vi "Keithley 2400 Source Measuret.vi"(8 "error in (no error)":errorcluster, 10 "Source Settings (Current vs Voltage Source)":T1(ring), 11 "VISA Refnum in":refnum<visa-resource-name>) -> (0 "error out":errorcluster, 3 "Source Value":dbl)   [LabVIEW 2019]
panel:
  # "This gets the value that the source is set\nat from the Keithley 2400\n\nJustin Young\n2012.06.24"
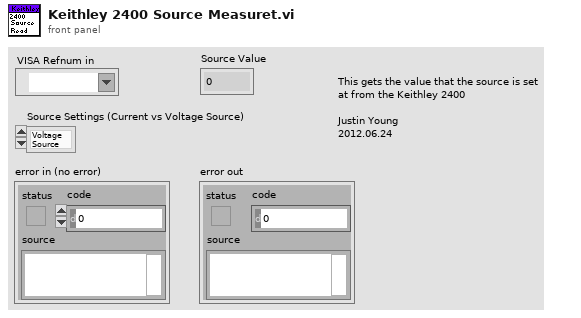
[diagram p1: front panel]
types:
  T1 = enum32{"Voltage Source", "Current Source", "Sense Only"}
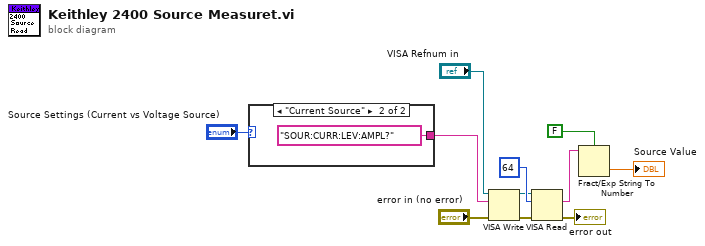
[diagram p0: block diagram]
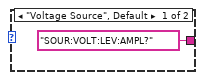
[diagram p2: hidden frame]
diagram:
  n1 = case shown="\"Current Source\"" "Source Settings (Current vs Voltage Source)" {
    tunnel: ["SOUR:VOLT:LEV:AMPL?" ("write buffer") "SOUR:CURR:LEV:AMPL?" ("write buffer")] -> w7
    frame "Voltage Source", Default {
    }
    frame "Current Source" {
    }
  }
  n2 = VISA Write(VISA resource name="VISA Refnum in", write buffer=w7, error in (no error)="error in (no error)") -> (VISA resource name out=w4:refnum<visa-resource-name>, error out=w3:errorcluster)  [unwired: 1 out]
  n3 = VISA Read(VISA resource name=w4, byte count=u32 64, error in (no error)=w3) -> (read buffer=w8:string, error out=→"error out":errorcluster)  [unwired: 2 out]
  n4 = Fract/Exp String To Number(use system decimal point (T)=FALSE, string=w8) -> (number=→"Source Value":dbl)  [unwired: 2 in, 1 out]
